vi "create module v2.vi"(7 "pClientData":u32, 8 "error in (no error)":errorcluster, 9 "p":dbl, 10 "zName":string, 11 "db":dbl) -> (0 "error out":errorcluster, 2 "function return":i32, 3 "db out":dbl, 5 "pClientData out":u32)   [LabVIEW 2020, in "sqlite3.lvlib"]
uses:
  sqlite3.lvlib
  errstr.vi
  bin/sqlite3_64.dll
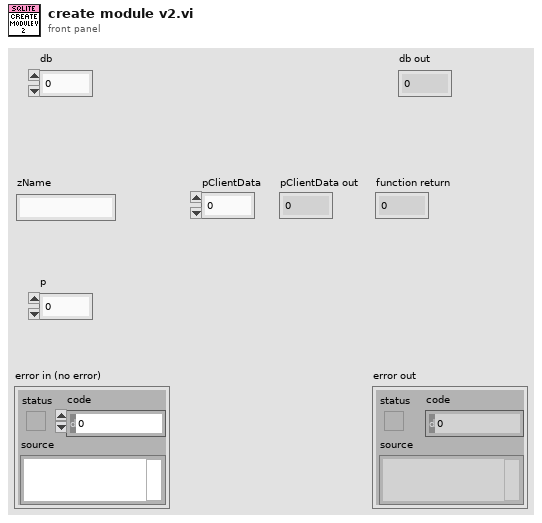
[diagram p1: front panel]
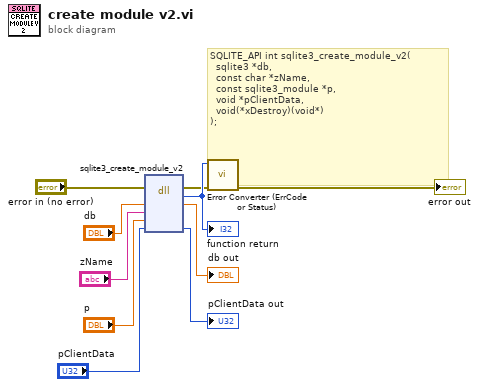
[diagram p0: block diagram]
diagram:
  # "SQLITE_API int sqlite3_create_module_v2(\n  sqlite3 *db,               \n  const char *zName,         \n  const sqlite3_module *p,   \n  void *pClientData,         \n  void(*xDestroy)(void*)     \n);"
  n1 = dll-call lib="C:/Users/Fred.Guo/Desktop/Database-configuration/externals/sqlite3/Source/bin/sqlite3_*.*" fn="sqlite3_create_module_v2"(error in="error in (no error)", "db"="db", "zName"="zName", "p"="p", "pClientData"="pClientData") -> (error out=w2:errorcluster, w10:i32, "db"=→"db out":dbl, "pClientData"=→"pClientData out":u32)  [unwired: 4 in, 1 out]
  "function return" <- w10
  n2 = call "Error Converter (ErrCode or Status).vi"("error in (no error)"=w2, "error code"=w10) -> ("error out"=→"error out":errorcluster)  [unwired: 9 in]
